vi "Delete All.vi"(0 "Display State In":T1={"Panels_Refnums_Array"=[], "Panel_Command"={"Operation"=enum."Add Item", "Data"=variant}}, 9 "Container State":T4, 11 "error in (no error)":errorcluster) -> (4 "Display State Out":T1={"Panels_Refnums_Array"=[], "Panel_Command"={"Operation"=enum."Add Item", "Data"=variant}}, 15 "error out":errorcluster)   [LabVIEW 2013, in "UI Panels.lvlib" / "Panels_XControl.xctl"]
uses:
  Panels_XControl.xctl
  <vilib>/_xctls/Container State.ctl
  State 1.ctl
  Controls/References/Panel_Refnums.ctl
  Controls/Panel_Command_Enum.ctl
  <vilib>/_xctls/XControlSupport.lvlib
panel:
  # "Delete All Panels Method No controls required."
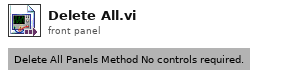
[diagram p1: front panel]
types:
  T1 = typedef "UI Panels.lvlib/Panels_XControl.xctl/State 1.ctl" = cluster{"Panels_Refnums_Array":T2[], "Panel_Command":cluster{"Operation":T3, "Data":variant}}
  T2 = typedef "UI Panels.lvlib/Panels_XControl.xctl/Panel_Refnums.ctl" = cluster{"VI Refnum":refnum<vi>, "Command":refnum<user-event>, "Visible":bool}
  T3 = typedef "UI Panels.lvlib/Panels_XControl.xctl/Panel_Command_Enum.ctl" = enum16{"Idle", "Remove & Stop", "Add Item", "Delete Item", "Delete All", "Insert into Subpanel", "Register Menu Events", "Update Value", "Remove from Subpanel", "Set Title", "Set Menu Items", "Insert SubPanel", "Set Splitter Position", "Set Splitter Properties", "Add Menu Items"}
  T4 = typedef "XControlSupport.lvlib/Container State.ctl" = cluster{"Indicator?":bool, "Run Mode?":bool, " Refnum":refnum<vi>}
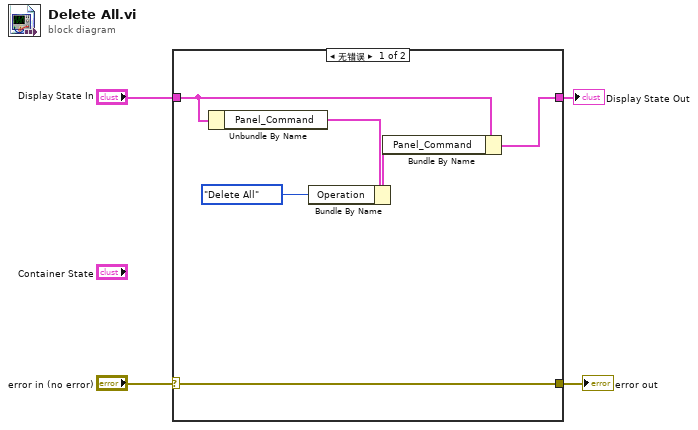
[diagram p0: block diagram]
diagram:
  n1 = case shown="无错误" "error in (no error)" {
    selector: "error in (no error)" -> [w7 w12]
    tunnel: "Display State In" -> [w6 w11]
    tunnel: [w8 w11] -> w3
    tunnel: [w7 w12] -> w1
    frame No Error {
      n2 = Unbundle By Name(w6) -> ("Panel_Command"=w5:cluster{"Operation":T3, "Data":variant})
      n3 = Bundle By Name(cluster=w5, "Operation"=Panel_Command_Enum."Delete All") -> (w9:cluster{"Operation":T3, "Data":variant})
      n4 = Bundle By Name(cluster=w6, "Panel_Command"=w9) -> (w8:T1)
    }
    frame Error {
    }
  }
  "Display State Out" <- w3
  "error out" <- w1
